vi "subvi.vi"(8 "cluster in":T1, 9 "Boolean 2":bool=TRUE, 10 "Numeric 2":i32, 11 "String":string) -> (2 "String 3":string, 3 "String 2":string)   [LabVIEW 2015]
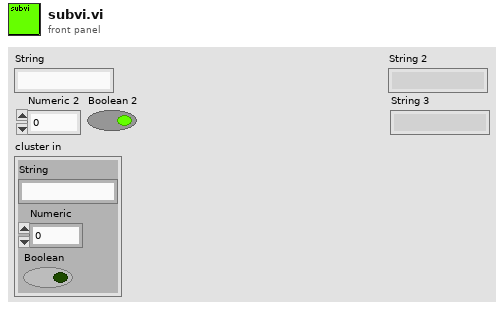
[diagram p1: front panel]
types:
  T1 = cluster{"String":string, "Numeric":i32, "Boolean":bool}
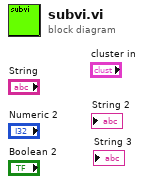
[diagram p0: block diagram]
diagram:
